vi "LoadConfiguration.vi"(0 "instruction target in":refnum<class "niInstr Instruction Target v1 Host.lvclass">, 1 "Configuration":T2[](array[typedef]), 5 "ScalingAndLimitsContext":refnum<class "niInstr Instruction Framework Context v1 Host.lvclass">, 11 "error in (no error)":errorcluster) -> (4 "Interface":T1, 15 "error out":errorcluster)   [LabVIEW 2017, in "ScaleAndLimitInterface.lvlib"]
uses:
  ScaleAndLimitInterface.lvlib
  Configuration.ctl
  <instrlib>/_niInstr/Instruction Framework/v1/Host/Instruction Framework Context/niInstr Instruction Framework Context v1 Host.lvclass
  Interface.ctl
  <instrlib>/_niInstr/Instruction Framework/v1/Host/Instruction Target/niInstr Instruction Target v1 Host.lvclass
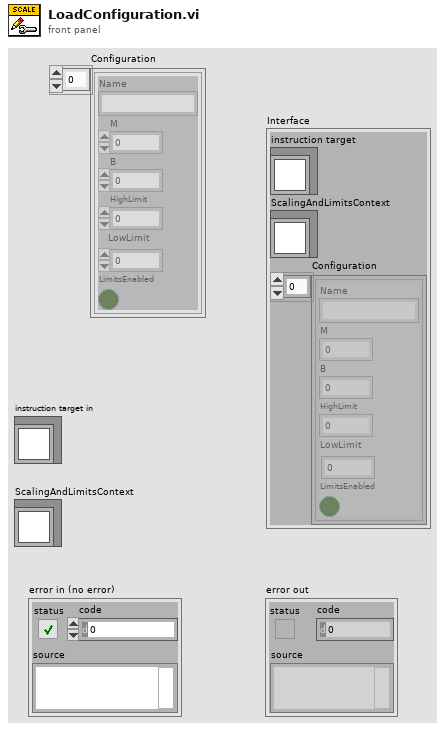
[diagram p1: front panel]
types:
  T1 = typedef "ScaleAndLimitInterface.lvlib/Interface.ctl" = cluster{"instruction target":refnum<class "niInstr Instruction Target v1 Host.lvclass">, "ScalingAndLimitsContext":refnum<class "niInstr Instruction Framework Context v1 Host.lvclass">, "Configuration":T2[]}
  T2 = typedef "ScaleAndLimitInterface.lvlib/Configuration.ctl" = cluster{"Name":string, "M":dbl, "B":i16, "HighLimit":dbl, "LowLimit":dbl, "LimitsEnabled":bool}
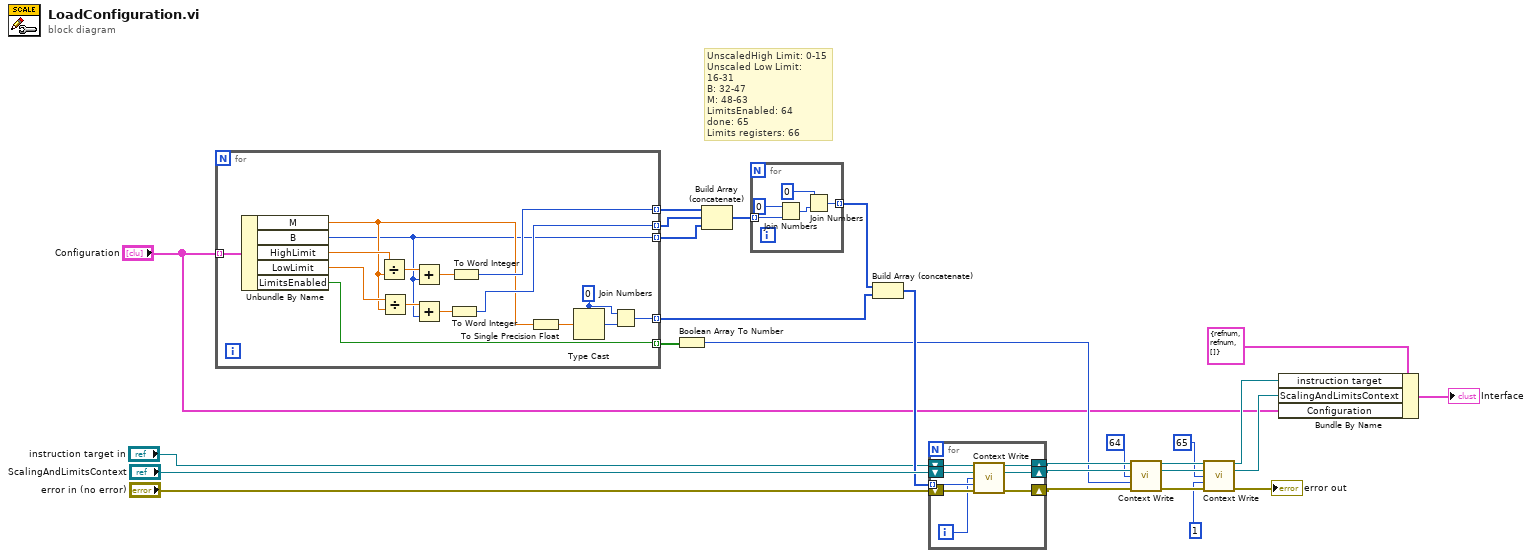
[diagram p0: block diagram]
diagram:
  # "UnscaledHigh Limit: 0-15\nUnscaled Low Limit: 16-31\nB: 32-47\nM: 48-63\nLimitsEnabled: 64\ndone: 65\nLimits registers: 66"
  n1 = for {
    tunnel: "Configuration" -> [w43] mode=indexing
    tunnel: [w36] -> w25 mode=indexing
    tunnel: [w35] -> w24 mode=indexing
    tunnel: [w33] -> w14 mode=indexing
    tunnel: [w29] -> w20 mode=indexing
    tunnel: [w28] -> w23 mode=indexing
    w30 = u32 0
    n2 = Unbundle By Name(w43) -> ("M"=w34:dbl, "B"=w28:i16, "HighLimit"=w42:dbl, "LowLimit"=w41:dbl, "LimitsEnabled"=w33:bool)
    n3 = Divide(x=w42, y=w34) -> (x/y=w39:dbl)
    n4 = Divide(x=w41, y=w34) -> (x/y=w40:dbl)
    n5 = Add(x=w39, y=w28) -> (x+y=w38:dbl)
    n6 = Add(x=w40, y=w28) -> (x+y=w37:dbl)
    n7 = To Word Integer(number=w37) -> (16bit integer=w35:i16)
    n8 = To Word Integer(number=w38) -> (16bit integer=w36:i16)
    n9 = To Single Precision Float(number=w34) -> (single precision float=w32:sgl)
    n10 = Type Cast(type=w30, x=w32) -> (*(type *) &x=w31:u32)
    n11 = Join Numbers(hi=w30, lo=w31) -> ((hi.lo)=w29:u64)
  }
  n12 = Boolean Array To Number(Boolean array=w14) -> (number=w13:u16)
  n13 = Build Array (concatenate)(w25, w24, w23) -> (w22:i16[])
  n14 = for {
    tunnel: w22 -> [w48] mode=indexing
    tunnel: [w44] -> w21 mode=indexing
    n15 = Join Numbers(hi=u16 0, lo=w48) -> ((hi.lo)=w46:u32)
    n16 = Join Numbers(hi=u32 0, lo=w46) -> ((hi.lo)=w44:u64)
  }
  n17 = Build Array (concatenate)(w21, w20) -> (w19:u64[])
  n18 = for {
    tunnel: w19 -> [w53] mode=indexing
    shift-right: [w51] -> w18
    shift-left: "instruction target in" -> [w54]
    shift-right: [w50] -> w17
    shift-left: "ScalingAndLimitsContext" -> [w56]
    shift-right: [w49] -> w16
    shift-left: "error in (no error)" -> [w55]
    i -> [w52]
    n19 = call <instrlib>:"Context Write.vi"("instruction target in"=w54, "context in"=w56, "address"=w52, "data"=w53, "error in"=w55) -> ("instruction target out"=w51:refnum<class "niInstr Instruction Target v1 Host.lvclass">, "context out"=w50:refnum<class "niInstr Instruction Framework Context v1 Host.lvclass">, "error out"=w49:errorcluster)  [unwired: 8 in]
  }
  n20 = call <instrlib>:"Context Write.vi"("instruction target in"=w18, "context in"=w17, "address"=u64 64, "data"=w13, "error in"=w16) -> ("instruction target out"=w12:refnum<class "niInstr Instruction Target v1 Host.lvclass">, "context out"=w11:refnum<class "niInstr Instruction Framework Context v1 Host.lvclass">, "error out"=w10:errorcluster)  [unwired: 8 in]
  n21 = call <instrlib>:"Context Write.vi"("instruction target in"=w12, "context in"=w11, "address"=u64 65, "data"=u64 1, "error in"=w10) -> ("instruction target out"=w5:refnum<class "niInstr Instruction Target v1 Host.lvclass">, "context out"=w4:refnum<class "niInstr Instruction Framework Context v1 Host.lvclass">, "error out"=→"error out":errorcluster)  [unwired: 8 in]
  n22 = Bundle By Name(cluster=T1 {"instruction target"=refnum, "ScalingAndLimitsContext"=refnum, "Configuration"=[]} ("Interface"), "instruction target"=w5, "ScalingAndLimitsContext"=w4, "Configuration"="Configuration") -> (→"Interface":T1)
